vi "Sleep Until FT External Clock.vi"(8 "error in (no error)":errorcluster, 10 "Wake Time":i64, 11 "CIFCorePlugin in":refnum<class "CIFCorePlugin.lvclass">) -> (0 "error out":errorcluster, 1 "Wake for Houskeeping":bool, 2 "Wake Time (ns)":i64, 3 "CIFCorePlugin out":refnum<class "CIFCorePlugin.lvclass">)   [LabVIEW 2021, in "CIFCorePlugin.lvclass"]
doc: "Sleep until a future time based on an external clock."
uses:
  CIFCorePlugin.lvclass
  CIFCorePlugin.lvclass/CIFCorePlugin.ctl
  Common/Typedef/Errors.ctl
  <vilib>/CIF Foundation/CIF Utilities/Time/System Time/LabVIEW Time to TAI Time.vi
  <vilib>/CIF Foundation/CIF Utilities/Errors/Append Error Location.vi
  Common/CIFCoreCommon.lvlib
  <vilib>/CIF Foundation/CIF Utilities/Time/Time_CIF_U.lvlib
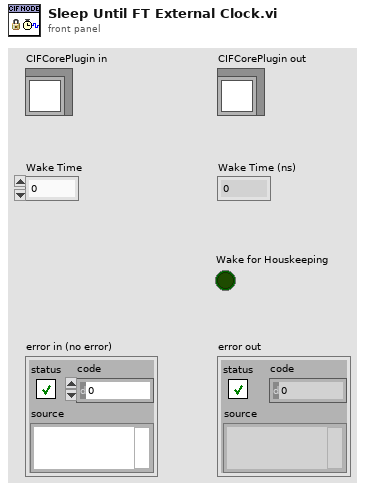
[diagram p1: front panel]
types:
  T1 = typedef "CIFCoreCommon.lvlib/Errors.ctl" = enum16{"Invalid Clock ID", "Long Sleep", "gRPC Server Not Found", "Config Parse", "Timestamp Wrap", "Delayed Execution", "Duplicate Channel", "Missing Channel", "Incorrect Type", "Flatten Error", "Unflatten Data", "Unique Name", "Plugin Not Found", "Plugin Type Not Found", "Plugin Version Not Found", "Manager Not Found", "Numerical Issue", "Time Jump", "Clock ID Match", "Channel Length", "Plugin Connection", "gRPC Server Connection", "PPL Name Match", "Build", "Config Log Parse", "Plugin Load", "UI Subpanel Load", "Python Name", "Invalid Name", "Unable to Change Ch Buffer"}
  T2 = typedef "Time_CIF_U.lvlib/Future Time Event Limits.ctl" = cluster{"Maximum":i64, "Minimum":i64}
  T3 = typedef "Time_CIF_U.lvlib/Clock Conversion Map.ctl" = map{u8, cluster{"Last Reset":i64, "Offset Pair":T4, "Slope":dbl, "1/Slope":dbl}}
  T4 = typedef "Time_CIF_U.lvlib/Timestamp Pair.ctl" = cluster{"System Time":i64, "External Time":i64}
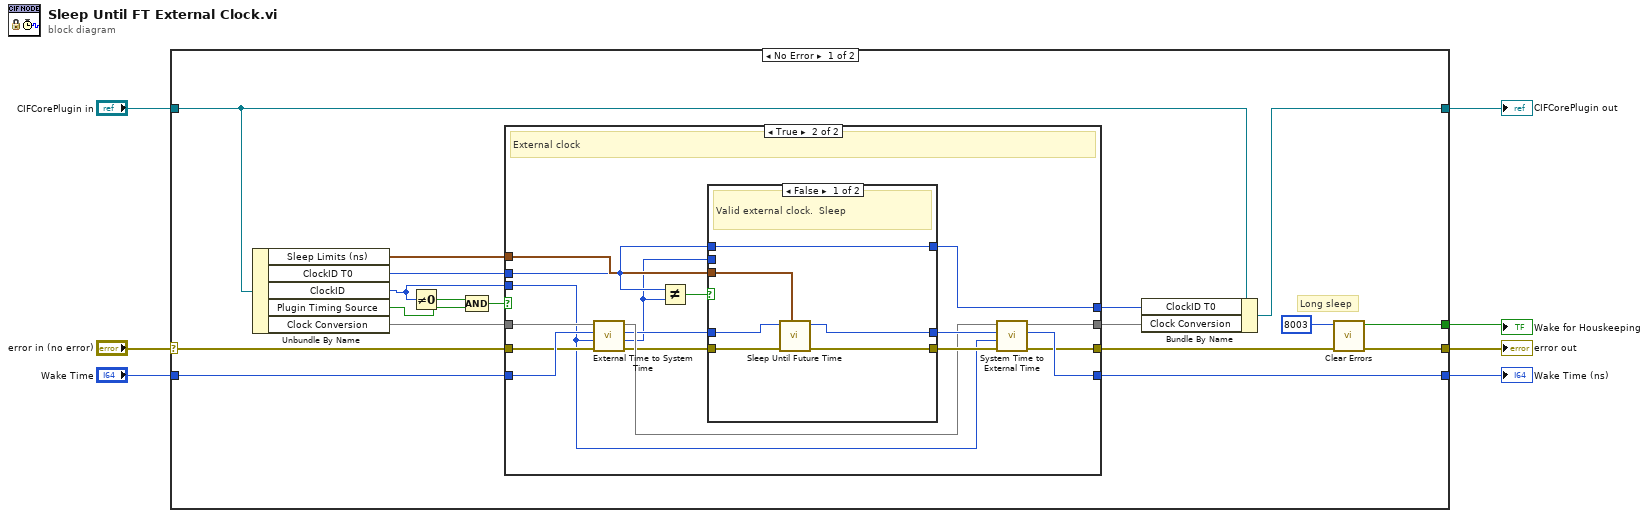
[diagram p0: block diagram]
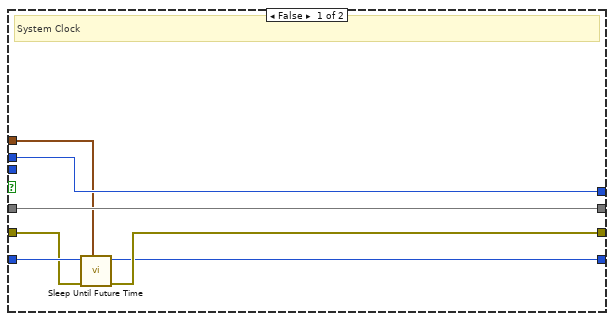
[diagram p2: hidden frame]
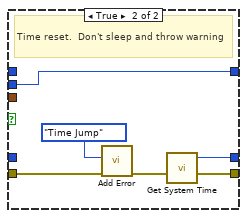
[diagram p3: hidden frame]
diagram:
  n1 = case shown="No Error" "error in (no error)" {
    selector: "error in (no error)" -> [w23 w62]
    tunnel: [w12 w62] -> w6
    tunnel: [w15 w61] -> w4
    tunnel: "CIFCorePlugin in" -> [w19 w61]
    tunnel: "Wake Time" -> [w25 _]
    tunnel: [w14 _] -> w2
    tunnel: [w13 _] -> w1
    frame No Error {
      # "Long sleep"
      n2 = Unbundle By Name(w19) -> ("Sleep Limits (ns)"=w20:T2, "ClockID T0"=w22:i64, "ClockID"=w9:u8, "Plugin Timing Source"=w8:bool, "Clock Conversion"=w24:T3)
      n3 = Not Equal To 0?(x=w9) -> (x != 0?=w11:bool)
      n4 = Compound Arithmetic op=AND(w11, w8) -> (w10:bool)
      n5 = case shown="True" w10 {
        tunnel: w25 -> [w30 w42]
        tunnel: w22 -> [w32 w47]
        tunnel: w24 -> [w31 w43]
        tunnel: w23 -> [w29 w38]
        tunnel: [w26 w36] -> w14
        tunnel: [w28 w34] -> w16
        tunnel: w20 -> [w27 w48]
        tunnel: [w31 w35] -> w18
        tunnel: [w32 w46] -> w17
        tunnel: w9 -> [_ w33]
        frame False {
          # "System Clock"
          n6 = call <vilib>:"Sleep Until Future Time.vi"("FTE Limits (ns)"=w27, "error in (no error)"=w29, "Wake Time (ns)"=w30) -> ("error out"=w28:errorcluster, "Sleep TIme"=w26:i64)  [unwired: 6 in, 1 out]
        }
        frame True {
          # "External clock"
          n7 = call <vilib>:"External Time to System Time.vi"("error in (no error)"=w38, "ClockID"=w33, "External Time"=w42, "Clock Convert Map in"=w43) -> ("error out"=w37:errorcluster, "Last Reset Time"=w39:i64, "System Time"=w40:i64, "Clock Convert Map out"=w41:T3)  [unwired: 4 in]
          n8 = Not Equal?(x=w47, y=w39) -> (x != y?=w49:bool)
          n9 = case shown="False" w49 {
            tunnel: w37 -> [w52 w58]
            tunnel: w40 -> [w53 _]
            tunnel: w48 -> [w54 _]
            tunnel: [w51 w57] -> w44
            tunnel: [w50 w59] -> w45
            tunnel: w47 -> [w55 _]
            tunnel: w39 -> [_ w60]
            tunnel: [w55 w60] -> w46
            frame False {
              # "Valid external clock.  Sleep"
              n10 = call <vilib>:"Sleep Until Future Time.vi"("FTE Limits (ns)"=w54, "error in (no error)"=w52, "Wake Time (ns)"=w53) -> ("error out"=w51:errorcluster, "Sleep TIme"=w50:i64)  [unwired: 6 in, 1 out]
            }
            frame True {
              # "Time reset.  Don't sleep and throw warning"
              n11 = call <vilib>:"Add Error.vi"("error in (no error)"=w58, "Error"=Errors."Time Jump") -> ("error out"=w57:errorcluster)  [unwired: 9 in]
              n12 = call <vilib>:"Get System Time.vi"() -> ("Time (ns)"=w59:i64)  [unwired: 5 in]
            }
          }
          n13 = call <vilib>:"System Time to External Time.vi"("error in (no error)"=w44, "ClockID"=w33, "System Time"=w45, "Clock Convert Map in"=w41) -> ("error out"=w34:errorcluster, "External Time"=w36:i64, "Clock Convert Map out"=w35:T3)  [unwired: 4 in, 1 out]
        }
      }
      n14 = Bundle By Name(cluster=w19, "ClockID T0"=w17, "Clock Conversion"=w18) -> (w15:refnum<class "CIFCorePlugin.lvclass">)
      n15 = call <vilib>:"Clear Errors.vi"("error in (no error)"=w16, "specific error code to clear (0: all)"=8003 ("code")) -> ("error out"=w12:errorcluster, "specific error cleared?"=w13:bool)  [unwired: 4 in]
    }
    frame Error {
    }
  }
  "error out" <- w6
  "CIFCorePlugin out" <- w4
  "Wake Time (ns)" <- w2
  "Wake for Houskeeping" <- w1
